vi "fwd cheesy drive.vi"(4 "Loop Timer":i32=20, 6 "Time to stop":i32=300, 8 "Distance":dbl, 9 "Encoder Left":dbl, 10 "Encoder Right":dbl, 11 "Yaw":dbl) -> (0 "Finished distance":bool, 1 "Both finished":bool, 2 "Direction":dbl, 3 "Trottle":dbl)   [LabVIEW 2017]
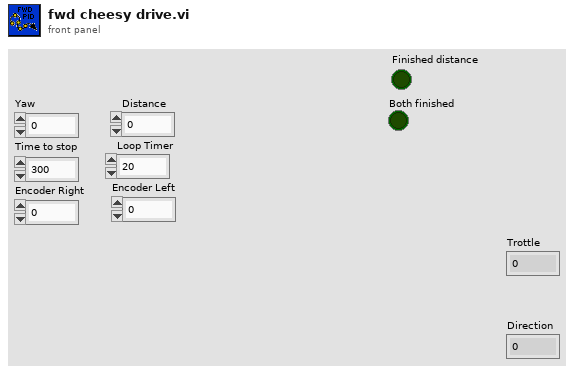
[diagram p1: front panel]
types:
  T1 = cluster{"proportional gain (Kc)":dbl, "integral time (Ti, min)":dbl, "derivative time (Td, min)":dbl}
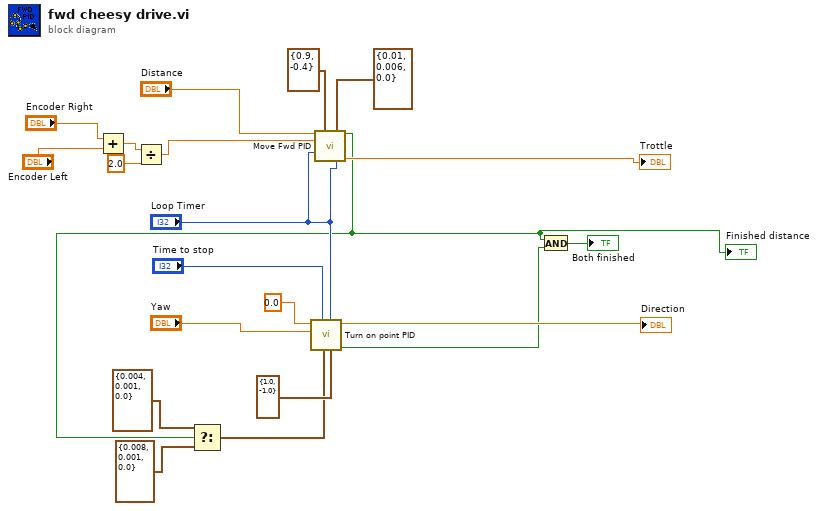
[diagram p0: block diagram]
diagram:
  n1 = Add(x="Encoder Right", y="Encoder Left") -> (x+y=w8:dbl)
  n2 = Divide(x=w8, y=2.0) -> (x/y=w6:dbl)
  n3 = call "Move Fwd PID.vi"("Distance"="Distance", "Range"=cluster{"output high":dbl, "output low":dbl} {"output high"=0.9, "output low"=-0.4}, "Gains"=T1 {"proportional gain (Kc)"=0.01, "integral time (Ti, min)"=0.006, "derivative time (Td, min)"=0.0}, "Encoder Count"=w6, "Time to stop"="Loop Timer", "Loop Timer"="Loop Timer") -> ("Finished?"=w1:bool, "Output"=→"Trottle":dbl)  [unwired: 8 in]
  "Finished distance" <- w1
  n4 = Select(t=T1 {"proportional gain (Kc)"=0.004, "integral time (Ti, min)"=0.001, "derivative time (Td, min)"=0.0} ("Gains"), s=w1, f=T1 {"proportional gain (Kc)"=0.008, "integral time (Ti, min)"=0.001, "derivative time (Td, min)"=0.0} ("Gains")) -> (s? t:f=w2:T1)
  n5 = call "Turn on point PID.vi"("Range"=cluster{"output high":dbl, "output low":dbl} {"output high"=1.0, "output low"=-1.0}, "Loop Timer"="Loop Timer", "Gains"=w2, "Time to stop"="Time to stop", "Yaw"="Yaw", "Setpoint(degrees)"=0.0) -> ("Finished?"=w5:bool, "PWM left"=→"Direction":dbl)  [unwired: 3 in, 1 out]
  n6 = And(x=w1, y=w5) -> (x .and. y?=→"Both finished":bool)
